vi "Type Conversion.To Double (1D Boolean).vi"(3 "values in":bool[](array[boolean])) -> (1 "values out":dbl[](array[numeric]))   [LabVIEW 2016, in "VeriStand Data.lvlib"]
doc: "Converts the provided values to double floats, preserving the numerical value of the data."
uses:
  VeriStand Data.lvlib
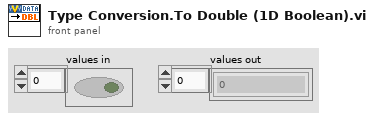
[diagram p1: front panel]
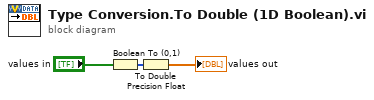
[diagram p0: block diagram]
diagram:
  n1 = Boolean To (0,1)(Boolean="values in") -> (0, 1=w2:i16[])
  n2 = To Double Precision Float(number=w2) -> (double precision float=→"values out":dbl[])
